vi "OP_Print_TPS20161121_cluster.vi"() -> ()   [LabVIEW 2013]
uses:
  <userlib>/caLab/Private/Get_PV-1D.vi
  <userlib>/caLab/Private/Get_PV.vi
panel:
  out "x = y?":bool
  out "NOW time":string
  out "NOW date":string
  out "loop2":i32=243
  in  "Save Button":bool
  out "error out 3":errorcluster
  in  "stop":bool
  out "time kickeron":string="kickers"
  out "date kickeron":string="wait to fire"
  out "Cluster":T1={"SR Fill Pattern"=array[864 elements], "Beam Current(mA"=301.91562200000004, "Beam Lifetime(min)"=669.1065769463743, "Beamsize X(um)"=55.54579477590784, "Beamsize Y(um)"=33.648665625479325, "Tune X(from BPM)"=0.1399, "Tune Y(from BPM)"=0.14, "Mode"="Top-Up", "NuX(from BBF) "=0.16718639681347974, "NuY(from BBF)"=0.25219386232318686, "IU22-23gap(R)"=11.0, "IU22-05gap(R)"=7.558, "IU22-05M"=TRUE, "IU22A-09gap(R)"=8.075, "IU22A-09M"=TRUE, "IU22B-09gap(R)"=40.001, "IU22B-09M"=FALSE, "IUT22-21gap(R)"=7.0, "IUT22-21M"=TRUE, "IU22-23M"=TRUE, "IU22A-25gap(R)"=8.18, "IU22A-25M"=TRUE, "IU22B-25gap(R)"=40.0, "IU22B-25M"=FALSE, "EPU48A-41gap(R)"=64.99985000000001, "EPU48A-41gM"=TRUE, "EPU48B-41gap(R)"=65.00399999999999, "EPU48B-41gM"=FALSE, "EPU46-45gap(R)"=45.00005, "EPU46-45gM"=TRUE, "EPU48A-41phase(R)"=0.0001, "EPU48B-41phase(R)"=0.00055, "EPU46-45phase(R)"=0.0, "Grid volt.(V)(S)"=33.0, "Gun mode"="MBM", "Mod.3 HV(kV)(S)"=35.800000000000026, "SR"="SR_DMB_2016_1102_1124LOCO.data", "BR"="Booster_JT_2016_1005_1200.data", "Linac"="Linac2016_1005_0935.data", "LTB"="LTB_JT_2016_1005_1200.data", "BTS"="BTS_2016_1116_1020.data", "RF2 remote"=TRUE, "RF2 OP mode"=TRUE, "RF2 phase.(S)"=-56.70000000000001, "RF Freq.(s)"=499654660.62238467, "RF2 gap volt.(S)"=1400.0, "RF3 remote"=TRUE, "RF3 OP mode"=TRUE, "RF3 phase.(S)"=160.0, "RF3 gap volt.(S)"=1400.0, "BBF V"=TRUE, "BBF H"=TRUE, "BR ext. kicker1(kV)"=18.266, "BR ext. kicker2(kV)"=18.26600000000001, "BR ext. sep.1(V)"=318.8444, "BR ext. sep.2(V)"=444.5, "BR inj. sep.(V)"=105.2, "BR inj. kicker(kV)"=16.40000000000001, "SR kicker4(kV)"=8.27, "SR kicker3(kV)"=8.315, "SR kicker2(kV)"=8.325, "SR kicker1(kV)"=8.4, "SR inj. sep.2(V)"=417.0, "SR inj. sep.1(V)"=419.3416, "Bucket Start"=100.0, "Bucket Last"=630.0, "Bucket Step"=10.0, "Orbit ILK(P)"=TRUE, "IU22-05 Hutch Enable"=TRUE, "IU22A-09M Hutch Enable"=TRUE, "IUT22-21M Hutch Enable"=TRUE, "IU22-23M Hutch Enable"=FALSE, "IU22A-25M Hutch Enable"=TRUE, "EPU48A-41M Hutch Enable"=FALSE, "EPU46-45M Hutch Enable"=TRUE, "EPU46-45 FE Enable"=TRUE, "EPU48A-41 FE Enable"=FALSE, "IU22A-25 FE Enable"=TRUE, "IU22-23 FE Enable"=FALSE, "IUT22-21 FE Enable"=TRUE, "IU22A-09 FE Enable"=TRUE, "IU22-05 FE Enable"=TRUE, "EPU48A-41pM"=TRUE, "EPU48B-41pM"=FALSE, "EPU46-45pM"=FALSE, "Gun volt.(V)(S)"=23.5, "Width count"=30.0, "2ns step"=0.0, "10ps delay"=100.0, "phase shifter"=130.00060000000002, "Taper"=-1.0899999999999999, "05XBPMX 1"=115.877, "09XBPMX 1"=471.421, "21XBPMX 1"=612.331, "23XBPMX 1"=-46.736000000000004, "25XBPMX 1"=462.29900000000004, "41XBPMX 1"=364.139, "45XBPMX 1"=-164.196, "05XBPMY 1"=-62.875, "09XBPMY 1"=-23.034, "21XBPMY 1"=-27.449, "23XBPMY 1"=-89.72200000000001, "25XBPMY 1"=459.291, "41XBPMY 1"=-111.624, "45XBPMY 1"=-57.689, "FOFB H"="On", "FOFB V"="On", "time string"="21:36:25", "date"="2016/11/21", "date (last kicker ON)"="wait to fire", "time string (last kicker ON)"="", "BPMX Graph"={[1, 2, 3, 4, 5, 6, 7, 8, 9, 10, 11, 12, 13, 14, 15, 16, 17, 18, 19, 20, 21, 22, 23, 24, 25, 26, 27, 28, 29, 30, 31, 32, 33, 34, 35, 36, 37, 38, 39, 40, 41, 42, 43, 44, 45, 46, 47, 48, 49, 50, 51, 52, 53, 54, 55, 56, 57, 58, 59, 60, 61, 62, 63, 64, 65, 66, 67, 68, 69, 70, 71, 72, 73, 74, 75, 76, 77, 78, 79, 80, 81, 82, 83, 84, 85, 86, 87, 88, 89, 90, 91, 92, 93, 94, 95, 96, 97, 98, 99, 100, 101, 102, 103, 104, 105, 106, 107, 108, 109, 110, 111, 112, 113, 114, 115, 116, 117, 118, 119, 120, 121, 122, 123, 124, 125, 126, 127, 128, 129, 130, 131, 132, 133, 134, 135, 136, 137, 138, 139, 140, 141, 142, 143, 144, 145, 146, 147, 148, 149, 150, 151, 152, 153, 154, 155, 156, 157, 158, 159, 160, 161, 162, 163, 164, 165, 166, 167, 168, 169, 170, 171, 172, 173, 174], "1rst Value (number)"=[-31.198, -3.303, -73.172, -2.032, 86.386, -75.851, 71.519, -46.03, 6.824, -37.804, 68.275, -4.672, -223.404, -16.867, -6.964, -259.448, -62.697, 1.8880000000000001, 75.267, -92.668, 86.714, -30.843, 12.767, -107.398, -44.436, 161.126, 208.922, 211.488, -27.247, 79.489, 826.962, 470.705, -115.522, -41.497, 159.486, -54.261, -0.64, 42.641, -2.466, -143.394, -24.785, 138.912, -65.805, 42.325, 32.891, -7.298, -96.724, -31.725, 98.531, -80.64, 64.163, 94.83, -44.03, -163.192, 50.589, 46.669000000000004, -87.508, 78.479, 31.618000000000002, -17.077, -125.32600000000001, -3.845, 98.34100000000001, -39.679, 50.247, -58.208, 40.297000000000004, -69.857, 42.548, -19.403, -211.0, -9.082, -322.597, -233.847, -140.75, 97.087, -15.869, -29.053, 59.46, -115.316, 70.896, -60.685, 33.715, 12.09, -520.422, -138.423, -302.753, 79.862, 120.014, 122.671, -55.812, 27.084, 39.115, -138.936, 156.631, 53.777, -72.647, -52.588, 16.002, 45.197, -117.489, 121.709, 27.952, -31.609, -113.58500000000001, 45.019, 55.136, -130.553, 138.93200000000002, 35.998, -30.631, -96.529, -7.589, 100.395, -93.919, 40.569, 79.538, -68.044, -134.578, 2.52, 84.539, -59.166000000000004, 42.576, 34.657000000000004, -15.805, -52.158, 18.484, 4.346, -157.404, 182.672, 202.518, -164.868, -53.871, 8.066, -9.738, -55.594, 92.623, -13.785, 11.587, -60.627, -47.704, 65.516, 57.924, 148.347, -201.348, -302.753, 189.117, 72.681, -134.928, 39.791000000000004, 45.938, -49.072, 54.473, 28.991, -20.657, -80.283, -20.264, 106.907, -121.271, 150.281, -2.243, -11.844, -122.82300000000001, 0.973, 114.186, -107.94, 95.485, 40.314, -36.956, -134.537, 16.196, 91.88, -35.505, -0.018000000000000002]}, "BPMY Graph"={[1, 2, 3, 4, 5, 6, 7, 8, 9, 10, 11, 12, 13, 14, 15, 16, 17, 18, 19, 20, 21, 22, 23, 24, 25, 26, 27, 28, 29, 30, 31, 32, 33, 34, 35, 36, 37, 38, 39, 40, 41, 42, 43, 44, 45, 46, 47, 48, 49, 50, 51, 52, 53, 54, 55, 56, 57, 58, 59, 60, 61, 62, 63, 64, 65, 66, 67, 68, 69, 70, 71, 72, 73, 74, 75, 76, 77, 78, 79, 80, 81, 82, 83, 84, 85, 86, 87, 88, 89, 90, 91, 92, 93, 94, 95, 96, 97, 98, 99, 100, 101, 102, 103, 104, 105, 106, 107, 108, 109, 110, 111, 112, 113, 114, 115, 116, 117, 118, 119, 120, 121, 122, 123, 124, 125, 126, 127, 128, 129, 130, 131, 132, 133, 134, 135, 136, 137, 138, 139, 140, 141, 142, 143, 144, 145, 146, 147, 148, 149, 150, 151, 152, 153, 154, 155, 156, 157, 158, 159, 160, 161, 162, 163, 164, 165, 166, 167, 168, 169, 170, 171, 172, 173, 174], "1rst Value (number)"=[-99.743, 2.851, -30.024, 83.777, -46.733000000000004, -39.889, 2.349, -4.944, 17.022000000000002, 9.824, 11.632, 41.188, -13.992, 13.911, -6.211, 53.857, -48.993, -32.789, -6.3740000000000006, -62.867000000000004, -8.332, 72.09400000000001, -75.398, 53.283, 63.008, -2.23, 43.024, 32.073, -246.641, -93.162, 456.41700000000003, 88.299, 58.803000000000004, 1.7590000000000001, 35.664, 6.575, 18.59, -30.439, 11.254, -28.256, -62.707, -4.503, 1.31, -21.571, 34.77, -8.876, 31.237000000000002, 25.402, 2.726, 20.655, -7.845, -1.443, -31.935000000000002, -16.981, 13.022, 17.515, -82.867, 61.285000000000004, -57.573, 110.363, -27.753, 28.322, -9.241, 53.929, -25.816, 24.231, -57.876, -11.578, 32.087, -70.84, 64.43, 9.409, -157.639, -57.0, 39.267, 30.23, 18.993000000000002, -33.97, 26.195, -10.585, -17.617, -18.667, 31.615000000000002, -25.437, 29.564, 13.537, 6.728, 163.38400000000001, 106.51, -70.056, 12.874, -4.125, -10.855, -21.856, 1.947, 8.096, 11.402000000000001, 5.761, 41.929, -8.752, 18.634, 7.553, -40.034, 39.183, -25.067, -32.557, 5.393, -17.564, -1.614, 20.498, -14.818, 10.313, 35.254, -35.886, 58.359, -36.56, -20.354, 7.593, -21.256, -8.001, -16.79, 10.18, -16.327, 20.416, -10.539, 19.944, -6.801, 13.068, -13.644, 3.468, -0.983, -17.6, 6.785, -26.101, -11.52, 61.191, -32.777, 13.536, 4.026, -14.682, 52.057, -53.883, 27.118000000000002, 31.672, 79.62, 17.715, 15.693, 113.157, -57.095, 14.214, -4.787, -11.148, -3.157, -6.251, -0.764, 3.563, 7.3500000000000005, 10.779, 21.129, 11.36, 7.771, -14.787, -13.278, 0.279, -13.516, -62.422000000000004, -13.389000000000001, 80.56400000000001, -108.465, 69.885, 30.116, 21.421, 32.779, -10.527000000000001]}, "Radio Buttons 2"=enum."absolute"} {"45XBPMY 1" format="%#.2f"; "41XBPMY 1" format="%#.2f"; "25XBPMY 1" format="%#.2f"; "23XBPMY 1" format="%#.2f"; "21XBPMY 1" format="%#.2f"; "09XBPMY 1" format="%#.2f"; "05XBPMY 1" format="%#.2f"; "45XBPMX 1" format="%#.2f"; "41XBPMX 1" format="%#.2f"; "25XBPMX 1" format="%#.2f"; "23XBPMX 1" format="%#.2f"; "21XBPMX 1" format="%#.2f"; "09XBPMX 1" format="%#.2f"; "05XBPMX 1" format="%#.2f"; "Taper" format="%#.4f"; "phase shifter" format="%#.3f"; "10ps delay" format="%#.1f"; "2ns step" format="%#.1f"; "Width count" format="%#.1f"; "Gun volt.(V)(S)" format="%#.1f"; "Bucket Step" format="%#.2f"; "Bucket Last" format="%#.2f"; "Bucket Start" format="%#.2f"; "BR ext. kicker1(kV)" format="%#.2f"; "BR ext. kicker2(kV)" format="%#.2f"; "BR ext. sep.1(V)" format="%#.2f"; "BR ext. sep.2(V)" format="%#.2f"; "BR inj. sep.(V)" format="%#.3f"; "BR inj. kicker(kV)" format="%#.3f"; "SR kicker4(kV)" format="%#.2f"; "SR kicker3(kV)" format="%#.2f"; "SR kicker2(kV)" format="%#.2f"; "SR kicker1(kV)" format="%#.2f"; "SR inj. sep.2(V)" format="%#.2f"; "SR inj. sep.1(V)" format="%#.2f"; "RF3 gap volt.(S)" format="%#.0f"; "RF3 phase.(S)" format="%#.1f"; "RF2 gap volt.(S)" format="%#.0f"; "RF Freq.(s)" format="%#.1f"; "RF2 phase.(S)" format="%#.1f"; "Mod.3 HV(kV)(S)" format="%#.3f"; "Grid volt.(V)(S)" format="%#.1f"; "EPU46-45phase(R)" format="%#.4f"; "EPU48B-41phase(R)" format="%#.4f"; "EPU48A-41phase(R)" format="%#.4f"; "EPU46-45gap(R)" format="%#.4f"; "EPU48B-41gap(R)" format="%#.4f"; "EPU48A-41gap(R)" format="%#.4f"; "IU22B-25gap(R)" format="%#.4f"; "IU22A-25gap(R)" format="%#.4f"; "IUT22-21gap(R)" format="%#.4f"; "IU22B-09gap(R)" format="%#.4f"; "IU22A-09gap(R)" format="%#.4f"; "IU22-05gap(R)" format="%#.4f"; "IU22-23gap(R)" format="%#.4f"; "NuY(from BBF)" format="%#.4f"; "NuX(from BBF)" format="%#.4f"; "Tune Y(from BPM)" format="%#.4f"; "Tune X(from BPM)" format="%#.4f"; "Beamsize Y(um)" format="%#.2f"; "Beamsize X(um)" format="%#.2f"; "Beam Lifetime(min)" format="%#.3f"; "Beam Current(mA" format="%#.3f"}
  out "date (last Gun ON)":string="2016/08/29"
  out "time string (last Gun ON)":string="23:28:50"
  out "Value Array (number) 7":dbl[](array[numeric])=[115.877, -62.875, 471.421, -23.034, 612.331, -27.449, -46.736000000000004, -89.72200000000001, 462.29900000000004, 459.291, 364.139, -111.624, -164.196, -57.689]
  out "Value Array (number) 6":dbl[](array[numeric])=[7.558, 8.075, 40.001, 7.0, 11.0, 8.18, 40.0, 64.99985000000001, 0.0001, 65.00399999999999, 0.00055, 45.00005, 0.0, -1.0899999999999999, 130.00060000000002]
  out "1rst Value (string) 2":string[](array[string])=["MBM", "33", "23.5", "350", "35.8", "22485", "22485", "62", "30", "0", "0", "160", "100"]
  out "Value Array (number) 5":dbl[](array[numeric])=[499654641.19275105, 1.0, 0.0, 1335.005102558433, 1400.0, -56.1, 1.0, 0.0, 1362.1066276040413, 1400.0, 160.0]
  out "1rst Value (string)":string[](array[string])=["Linac2016_1005_0935.data", "LTB_JT_2016_1005_1200.data", "Booster_JT_2016_1005_1200.data", "BTS_2016_1116_1020.data", "SR_DMB_2016_1102_1124LOCO.data"]
  out "Value Array (number) 4":dbl[](array[numeric])=[499654660.62238467, 1.0, 0.0, 1334.266859115235, 1400.0, -56.70000000000001, 1.0, 0.0, 1364.570619451613, 1400.0, 160.0]
  out "Value Array (number) 3":dbl[](array[numeric])=[0.0, 33.0, 23.5, 350.0, 35.800000000000026, 22485.0, 22485.0, 62.0, 30.0, 0.0, 0.0, 160.0, 100.0]
  out "Value Array (number) 2":dbl[](array[numeric])=[105.2, 16.40000000000001, 18.266, 18.26600000000001, 318.8444, 444.5, 419.3416, 417.0, 8.4, 8.325, 8.315, 8.27]
  out "Value Array (number)":dbl[](array[numeric])=[1.0, 301.91562200000004, 669.1065769463743, 46.211143740355936, 27.993898190914578, 0.11937377690802348, 0.2162426614481409, 96.68439483642578, 145.84446716308594, 100.0, 630.0, 10.0]
  out "Orbit ILK(A)":bool
  out "Orbit INT. Ang Active":bool
  out "Orbit INT.Ang. On":bool
  out "Orbit INT. Pos Active":bool
  out "Orbit INT.Pos. On":bool
  out "SBM volt.(S)":dbl=350.0 format="%#.1f"
  out "MBM volt.(S)":dbl=23.5 format="%#.1f"
  in  "Copy Button":bool
  in  "Print Button":bool
  in  "Help Button":bool
  in  "Refresh Button":bool
  in  "Open Button":bool
  out "Gun WCM":dbl[](graph)
  out "BR Fill Pattern":dbl[](graph)
  # "TPS OP Handover Information"
  # "Others"
  # "Time："
  # "Valve  Status"
  # "SM Status"
  # "歷史電流圖\ntrip次數?\n輻射劑量?\n平均氣壓\n目前最高累計劑量\n最近一次觸發時BR電流及WCM數值"
  # "TPS Operational Handover Information v1.0"
  # "SR Status"
  # "Feedback"
  # "Pulse Mag"
  # "LINAC"
  # "x8(ns)"
  # "x2(ns)"
  # "x0.01(ns)"
  # "RF Status"
  # "Hz"
  # "(kV)"
  # "(kV)"
  # "Changeliang@LOP.NSRRC"
  # "SR Fill Pattern"
  # "Lattice Files in using"
  # "ID &Beamline (R)"
  # "Gap\nmm"
  # "Motor"
  # "Phase"
  # "FE/Hutch"
  # "phase\nshifter"
  # "Taper\n(enc)"
  # "XBPM1X\num"
  # "XBPM1Y\num"
  # "05"
  # "09"
  # "21"
  # "23"
  # "25"
  # "41"
  # "45"
  # "SR Orbit"
  # "BPMX"
  # "BPMY"
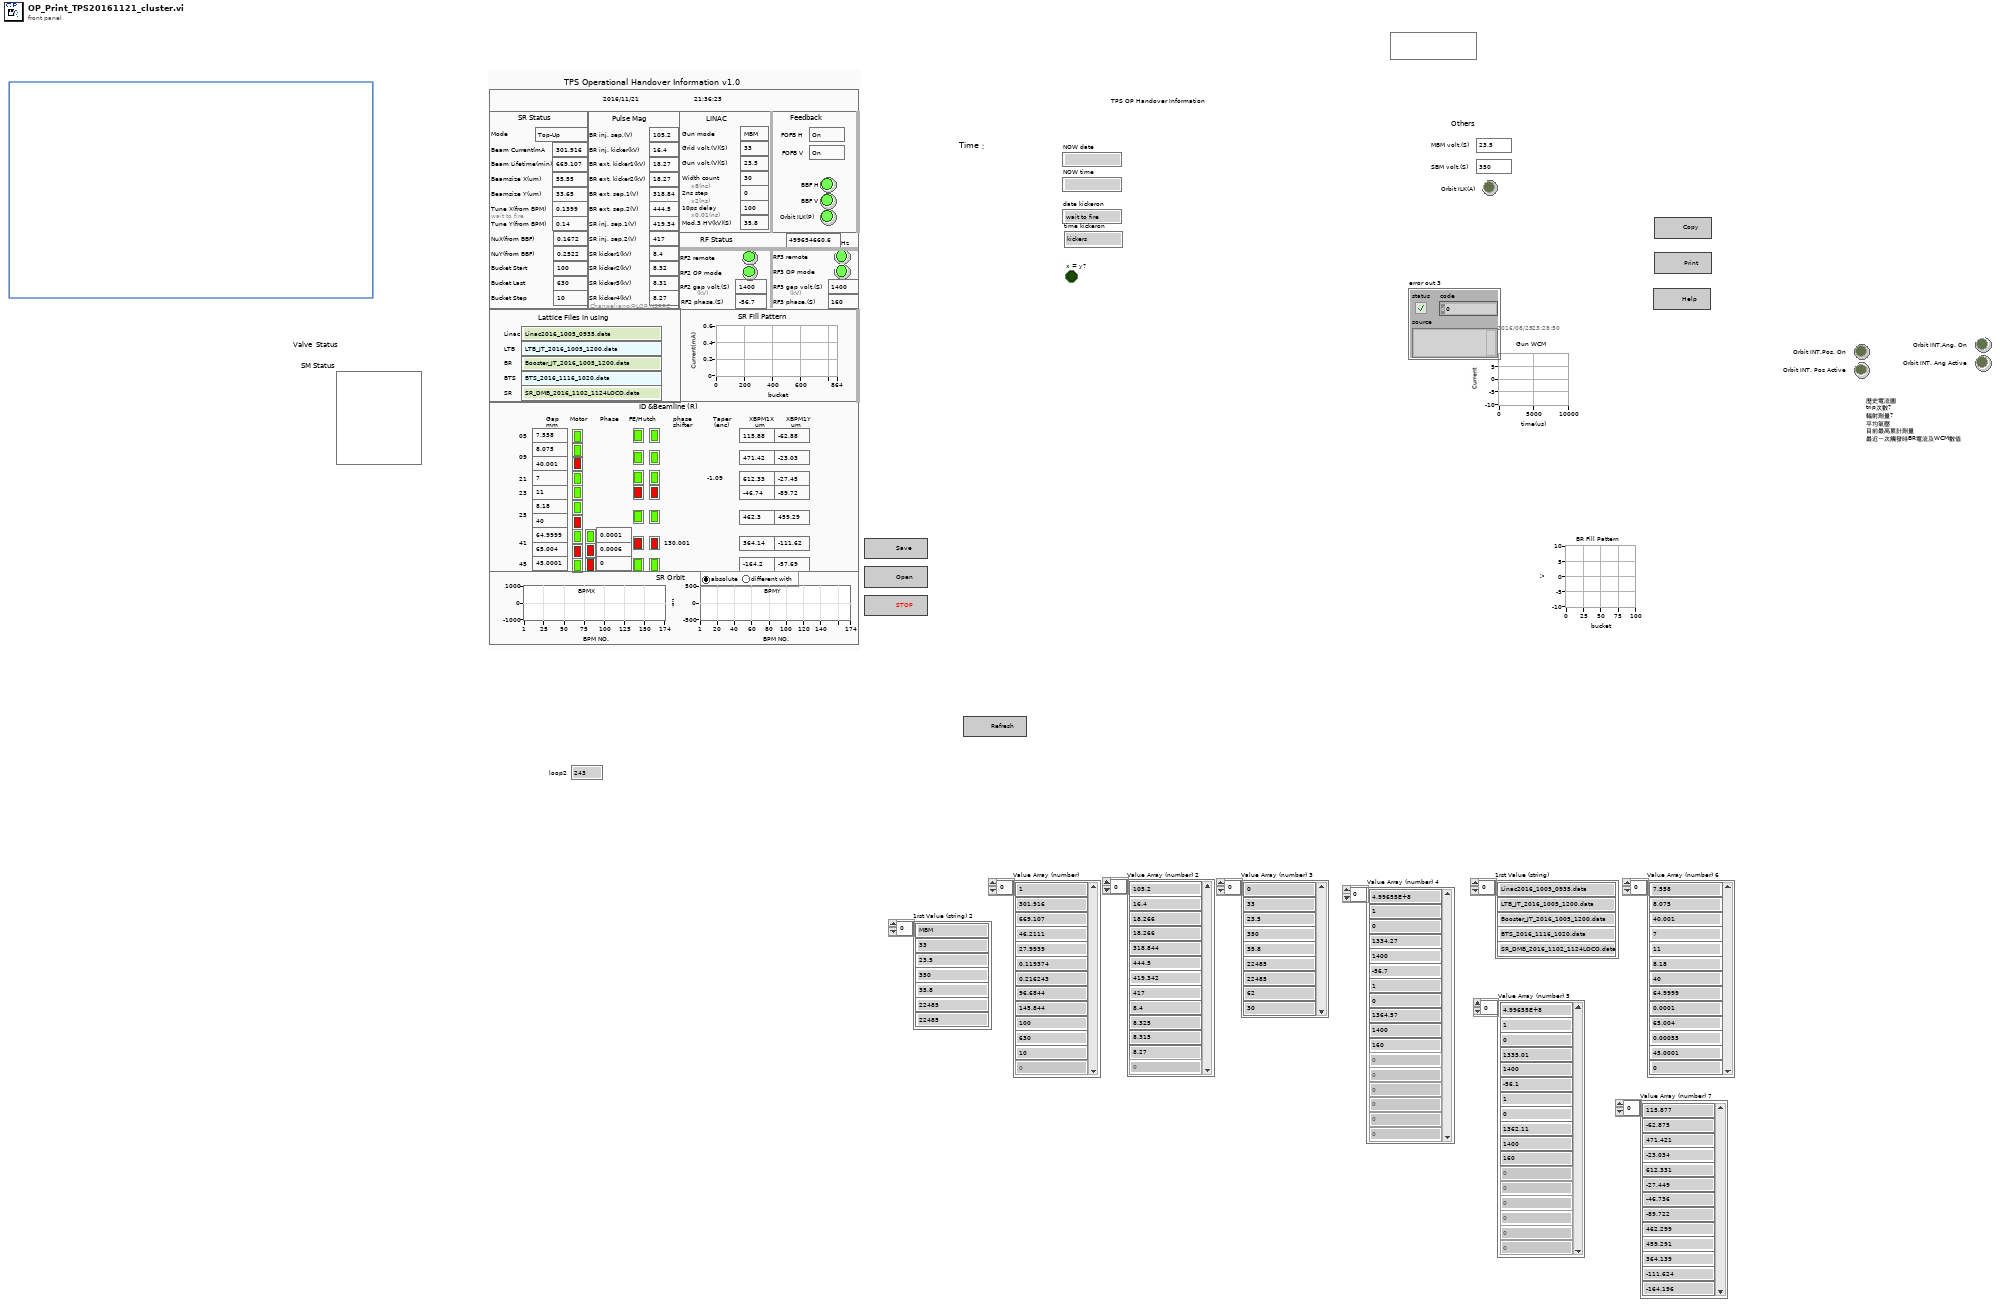
[diagram p1: front panel]
types:
  T1 = cluster{"SR Fill Pattern":dbl[], "Beam Current(mA":dbl, "Beam Lifetime(min)":dbl, "Beamsize X(um)":dbl, "Beamsize Y(um)":dbl, "Tune X(from BPM)":dbl, "Tune Y(from BPM)":dbl, "Mode":string, "NuX(from BBF) ":dbl, "NuY(from BBF)":dbl, "IU22-23gap(R)":dbl, "IU22-05gap(R)":dbl, "IU22-05M":bool, "IU22A-09gap(R)":dbl, "IU22A-09M":bool, "IU22B-09gap(R)":dbl, "IU22B-09M":bool, "IUT22-21gap(R)":dbl, "IUT22-21M":bool, "IU22-23M":bool, "IU22A-25gap(R)":dbl, "IU22A-25M":bool, "IU22B-25gap(R)":dbl, "IU22B-25M":bool, "EPU48A-41gap(R)":dbl, "EPU48A-41gM":bool, "EPU48B-41gap(R)":dbl, "EPU48B-41gM":bool, "EPU46-45gap(R)":dbl, "EPU46-45gM":bool, "EPU48A-41phase(R)":dbl, "EPU48B-41phase(R)":dbl, "EPU46-45phase(R)":dbl, "Grid volt.(V)(S)":dbl, "Gun mode":string, "Mod.3 HV(kV)(S)":dbl, "SR":string, "BR":string, "Linac":string, "LTB":string, "BTS":string, "RF2 remote":bool, "RF2 OP mode":bool, "RF2 phase.(S)":dbl, "RF Freq.(s)":dbl, "RF2 gap volt.(S)":dbl, "RF3 remote":bool, "RF3 OP mode":bool, "RF3 phase.(S)":dbl, "RF3 gap volt.(S)":dbl, "BBF V":bool, "BBF H":bool, "BR ext. kicker1(kV)":dbl, "BR ext. kicker2(kV)":dbl, "BR ext. sep.1(V)":dbl, "BR ext. sep.2(V)":dbl, "BR inj. sep.(V)":dbl, "BR inj. kicker(kV)":dbl, "SR kicker4(kV)":dbl, "SR kicker3(kV)":dbl, "SR kicker2(kV)":dbl, "SR kicker1(kV)":dbl, "SR inj. sep.2(V)":dbl, "SR inj. sep.1(V)":dbl, "Bucket Start":dbl, "Bucket Last":dbl, "Bucket Step":dbl, "Orbit ILK(P)":bool, "IU22-05 Hutch Enable":bool, "IU22A-09M Hutch Enable":bool, "IUT22-21M Hutch Enable":bool, "IU22-23M Hutch Enable":bool, "IU22A-25M Hutch Enable":bool, "EPU48A-41M Hutch Enable":bool, "EPU46-45M Hutch Enable":bool, "EPU46-45 FE Enable":bool, "EPU48A-41 FE Enable":bool, "IU22A-25 FE Enable":bool, "IU22-23 FE Enable":bool, "IUT22-21 FE Enable":bool, "IU22A-09 FE Enable":bool, "IU22-05 FE Enable":bool, "EPU48A-41pM":bool, "EPU48B-41pM":bool, "EPU46-45pM":bool, "Gun volt.(V)(S)":dbl, "Width count":dbl, "2ns step":dbl, "10ps delay":dbl, "phase shifter":dbl, "Taper":dbl, "05XBPMX 1":dbl, "09XBPMX 1":dbl, "21XBPMX 1":dbl, "23XBPMX 1":dbl, "25XBPMX 1":dbl, "41XBPMX 1":dbl, "45XBPMX 1":dbl, "05XBPMY 1":dbl, "09XBPMY 1":dbl, "21XBPMY 1":dbl, "23XBPMY 1":dbl, "25XBPMY 1":dbl, "41XBPMY 1":dbl, "45XBPMY 1":dbl, "FOFB H":string, "FOFB V":string, "time string":string, "date":string, "date (last kicker ON)":string, "time string (last kicker ON)":string, "BPMX Graph":cluster{i32[], "1rst Value (number)":dbl[]}, "BPMY Graph":cluster{i32[], "1rst Value (number)":dbl[]}, "Radio Buttons 2":enum32{"absolute", "different with"}}
  T2 = cluster{"SR Fill Pattern":dbl[], "Beam Current(mA":dbl, "Beam Lifetime(min)":dbl, "Beamsize X(um)":dbl, "Beamsize Y(um)":dbl, "Tune X(form BPM)":dbl, "Tune Y(form BPM)":dbl, "Mode":string, "NuX(form BBF) ":dbl, "NuY(form BBF)":dbl, "IU22-23gap(R)":dbl, "IU22-05gap(R)":dbl, "IU22-05M":bool, "IU22A-09gap(R)":dbl, "IU22A-09M":bool, "IU22B-09gap(R)":dbl, "IU22B-09M":bool, "IUT22-21gap(R)":dbl, "IUT22-21M":bool, "IU22-23M":bool, "IU22A-25gap(R)":dbl, "IU22A-25M":bool, "IU22B-25gap(R)":dbl, "IU22B-25M":bool, "EPU48A-41gap(R)":dbl, "EPU48A-41gM":bool, "EPU48B-41gap(R)":dbl, "EPU48B-41gM":bool, "EPU46-45gap(R)":dbl, "EPU46-45gM":bool, "EPU48A-41phase(R)":dbl, "EPU48B-41phase(R)":dbl, "EPU46-45phase(R)":dbl, "Grid volt.(S)":dbl, "Gun mode":string, "Mod.3 HV(S)":dbl, "SR":string, "BR":string, "Linac":string, "LTB":string, "BTS":string, "RF2 remote":bool, "RF2 OP mode":bool, "RF2 phase.(S)":dbl, "RF Freq.(s)":dbl, "RF2 gap volt.(S)":dbl, "RF3 remote":bool, "RF3 OP mode":bool, "RF3 phase.(S)":dbl, "RF3 gap volt.(S)":dbl, "BBF V":bool, "BBF H":bool, "BR ext. kicker1":dbl, "BR ext. kicker2":dbl, "BR ext. sep.1":dbl, "BR ext. sep.2":dbl, "BR inj. sep.":dbl, "BR inj. kicker":dbl, "SR kicker4":dbl, "SR kicker3":dbl, "SR kicker2":dbl, "SR kicker1":dbl, "SR inj. sep.2":dbl, "SR inj. sep.1":dbl, "Bucket Start":dbl, "Bucket Last":dbl, "Bucket Step":dbl, "Orbit ILK(P)":bool, "IU22-05 Hutch Enable":bool, "IU22A-09M Hutch Enable":bool, "IUT22-21M Hutch Enable":bool, "IU22-23M Hutch Enable":bool, "IU22A-25M Hutch Enable":bool, "EPU48A-41M Hutch Enable":bool, "EPU46-45M Hutch Enable":bool, "EPU46-45 FE Enable":bool, "EPU48A-41 FE Enable":bool, "IU22A-25 FE Enable":bool, "IU22-23 FE Enable":bool, "IUT22-21 FE Enable":bool, "IU22A-09 FE Enable":bool, "IU22-05 FE Enable":bool, "EPU48A-41pM":bool, "EPU48B-41pM":bool, "EPU46-45pM":bool, "Gun volt.(S)":dbl, "Width count":dbl, "2ns step":dbl, "10ps delay":dbl, "phase shifter":dbl, "Taper":dbl, "05XBPMX 1":dbl, "09XBPMX 1":dbl, "21XBPMX 1":dbl, "23XBPMX 1":dbl, "25XBPMX 1":dbl, "41XBPMX 1":dbl, "45XBPMX 1":dbl, "05XBPMY 1":dbl, "09XBPMY 1":dbl, "21XBPMY 1":dbl, "23XBPMY 1":dbl, "25XBPMY 1":dbl, "41XBPMY 1":dbl, "45XBPMY 1":dbl, "FOFB H":string, "FOFB V":string, "time string":string, "date":string, "date (last kicker ON)":string, "time string (last kicker ON)":string, "BPMX Graph":cluster{i32[], "1rst Value (number)":dbl[]}, "BPMY Graph":cluster{i32[], "1rst Value (number)":dbl[]}, "Radio Buttons 2":enum32{"absolute", "different with"}}
  T3 = typedef "imagedata.ctl" = cluster{"image type":i32, "image depth":i32, "image":u8[], "mask":u8[], "colors":u32[], "Rectangle":cluster{"left":i16, "top":i16, "right":i16, "bottom":i16}}
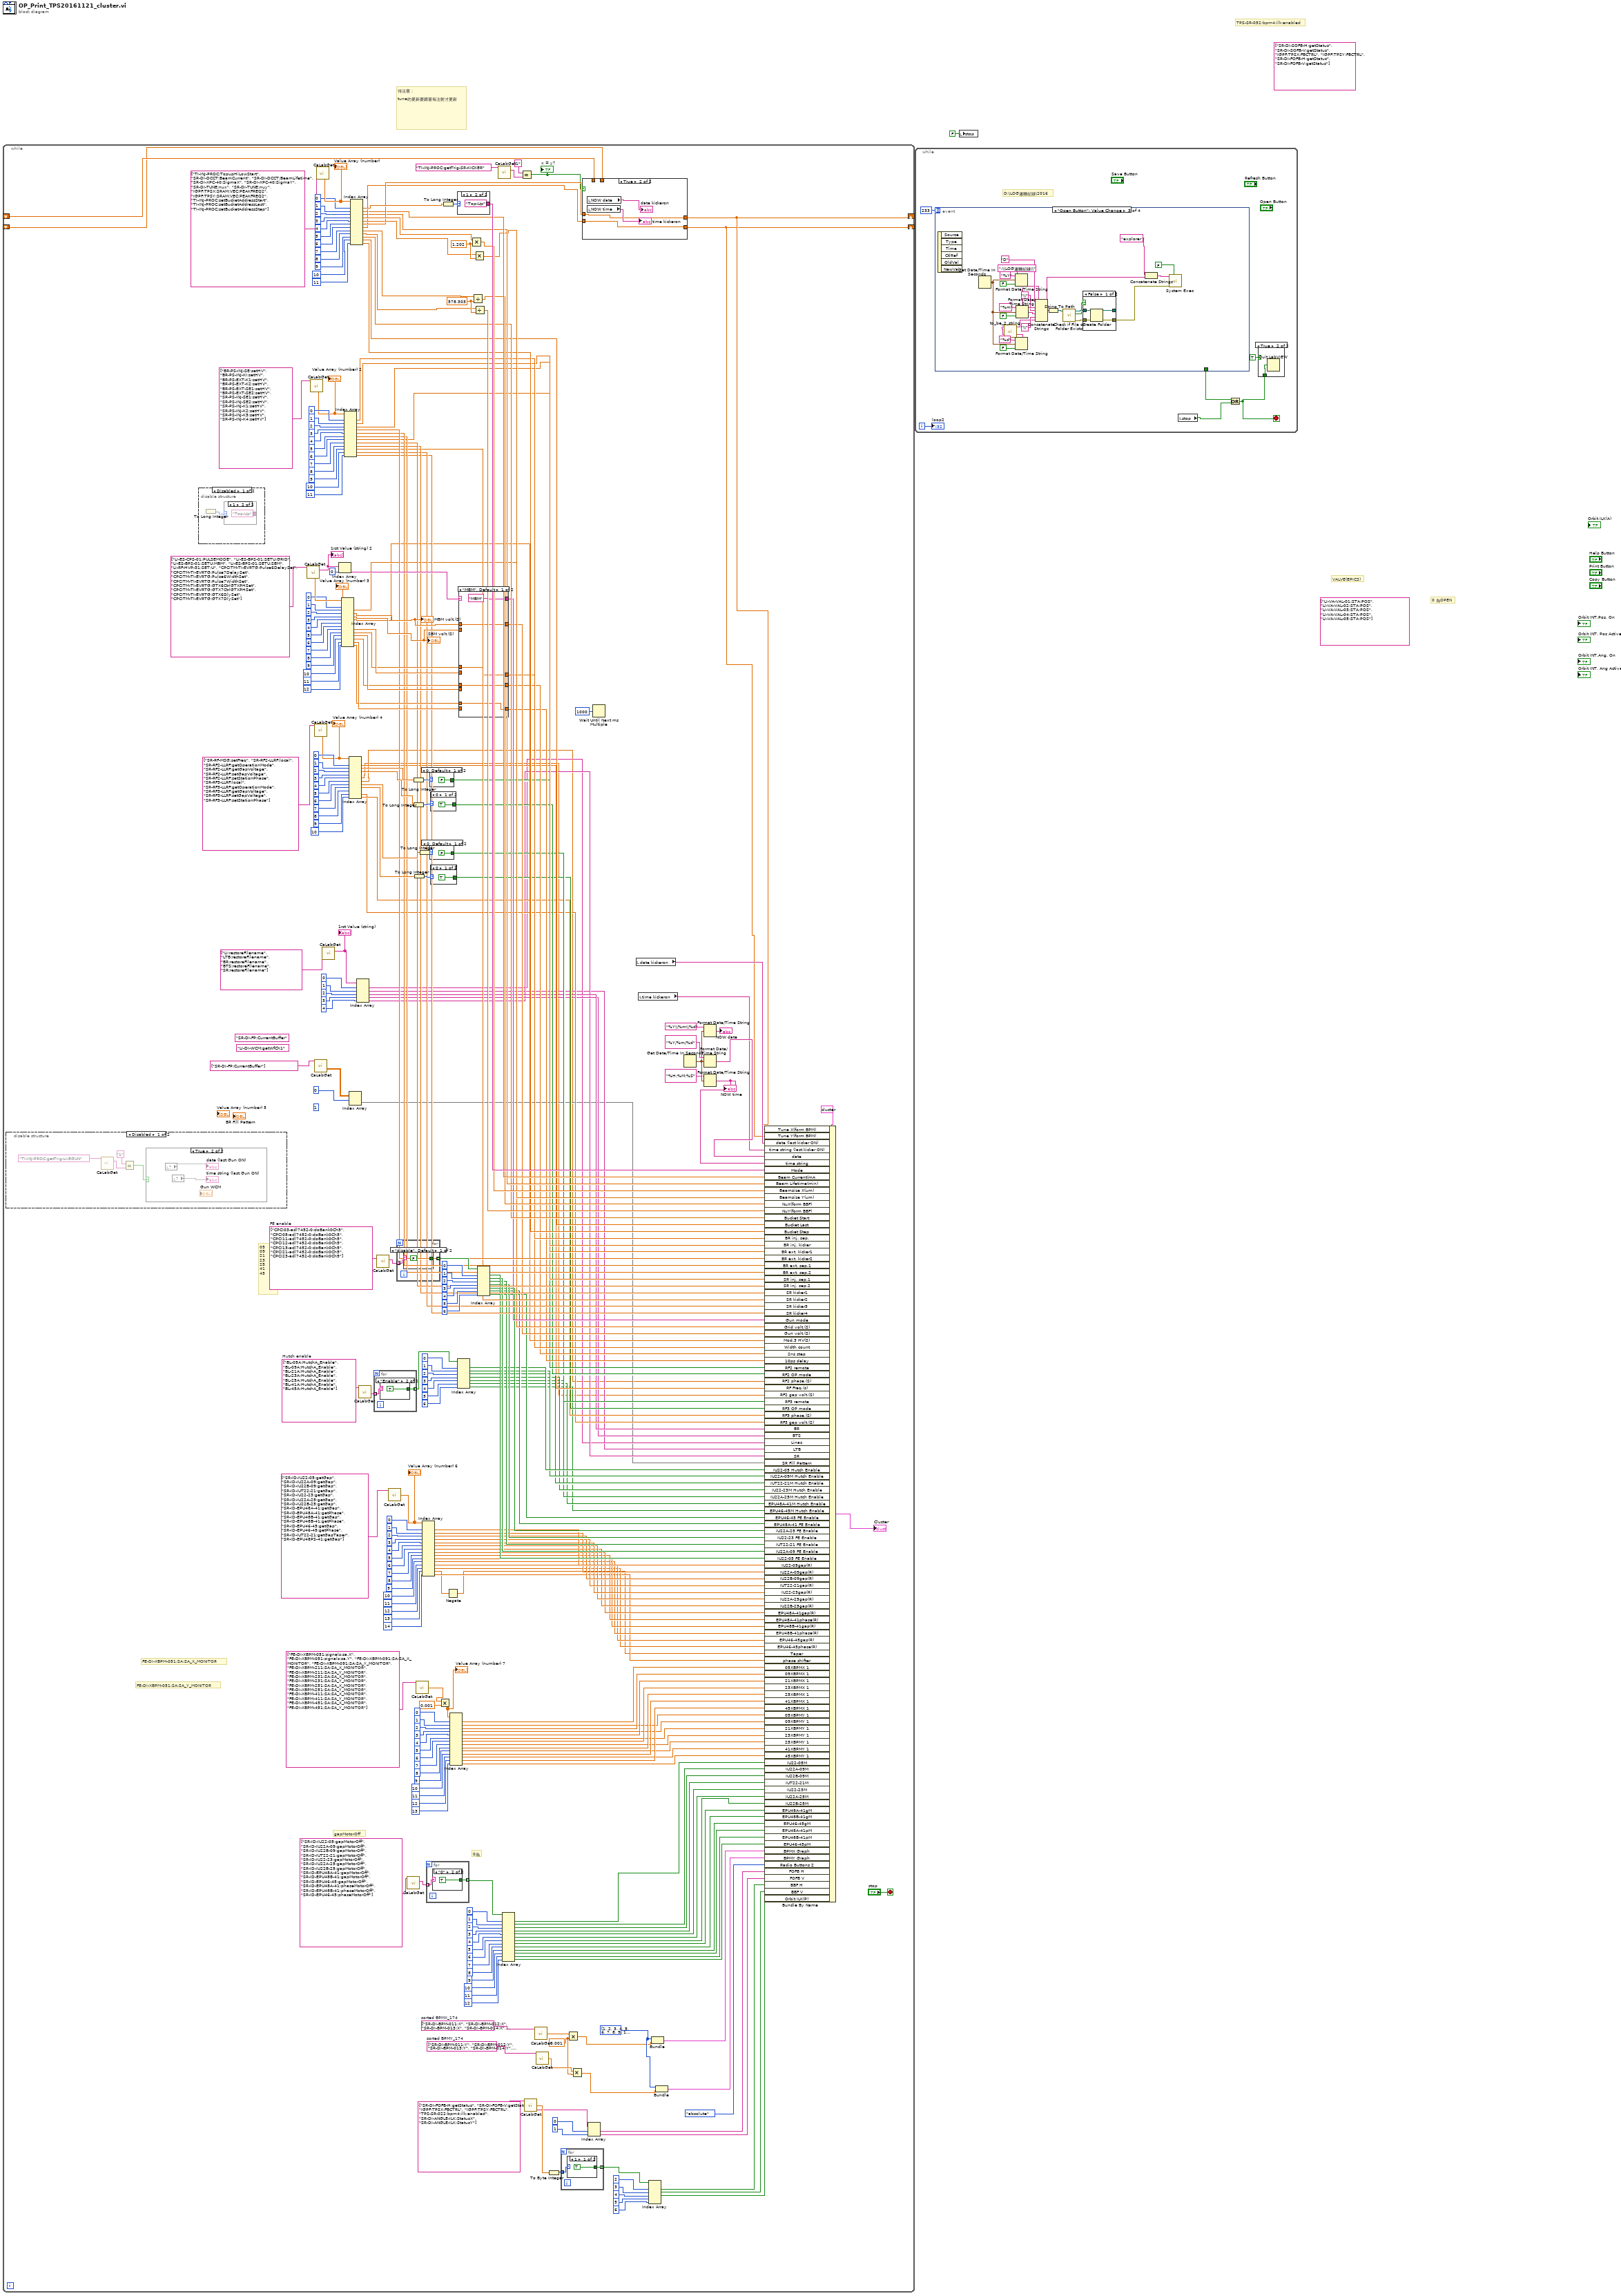
[diagram p0: block diagram]
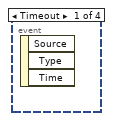
[diagram p3: hidden frame]
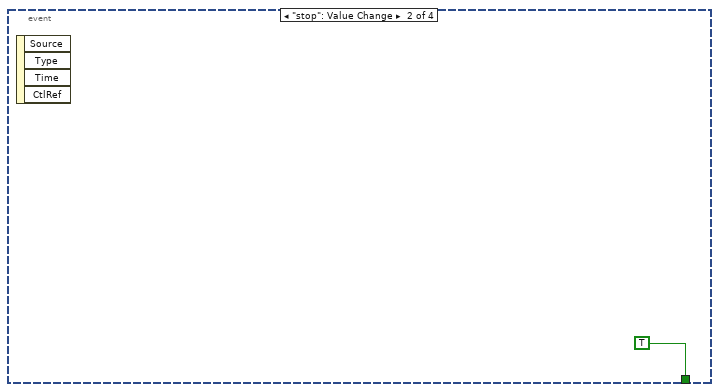
[diagram p4: hidden frame]
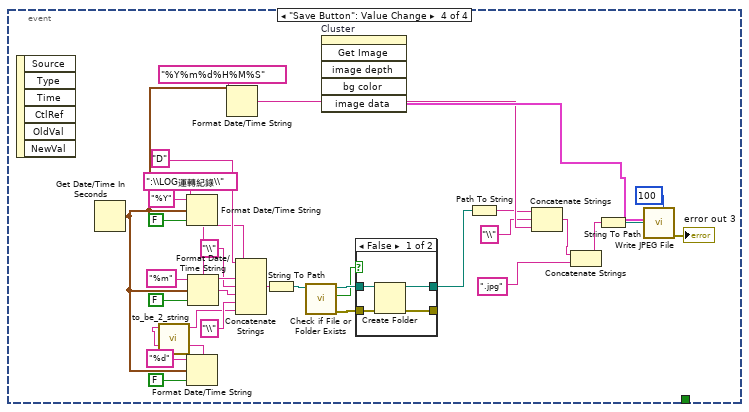
[diagram p6: hidden frame]
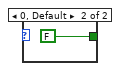
[diagram p8: hidden frame]
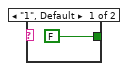
[diagram p11: hidden frame]
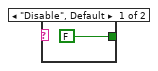
[diagram p12: hidden frame]
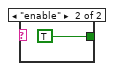
[diagram p13: hidden frame]
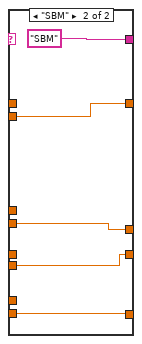
[diagram p14: hidden frame]
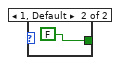
[diagram p16: hidden frame]
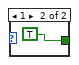
[diagram p17: hidden frame]
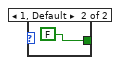
[diagram p18: hidden frame]
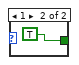
[diagram p19: hidden frame]
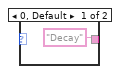
[diagram p20: hidden frame]
diagram:
  (unwired) string[] ["LI-VA-VAL-01:STA:POS", "LI-VA-VAL-02:STA:POS", "LI-VA-VAL-03:STA:POS", "LI-VA-VAL-04:STA:POS", "LI-VA-VAL-05:STA:POS"]
  (unwired) string[] ["SR-DI-SOFB-H:getStatus", "SR-DI-SOFB-V:getStatus", "IGPF:TPSX:FBCTRL", "IGPF:TPSY:FBCTRL", "SR-DI-FOFB-H:getStatus", "SR-DI-FOFB-V:getStatus"]
  # "TPS-SR-052:bpm4:ilk:enabled"
  # "待注意：\n\ntune的更新要跟著有注射才更新"
  # "0 為OPEN"
  # "VALVE(EPICS)"
  n1 = while {
    shift-right: [w5] -> _
    shift-left: _ -> [w3]
    shift-right: [w4] -> _
    shift-left: _ -> [w2]
    stop <- "stop" stop-if-true
    (unwired) "LI-DI-WCM:getWfCh1"
    (unwired) "SR-DI-FP:CurrentBuffer"
    w143 = i32[] [1, 2, 3, 4, 5, 6, 7, 8, 9, 10, 11, 12, 13, 14, 15, 16, 17, 18, 19, 20, 21, 22, 23, 24, 25, 26, 27, 28, 29, 30, 31, 32, 33, 34, 35, 36, 37, 38, 39, 40, 41, 42, 43, 44, 45, 46, 47, 48, 49, 50, 51, 52, 53, 54, 55, 56, 57, 58, 59, 60, 61, 62, 63, 64, 65, 66, 67, 68, 69, 70, 71, 72, 73, 74, 75, 76, 77, 78, 79, 80, 81, 82, 83, 84, 85, 86, 87, 88, 89, 90, 91, 92, 93, 94, 95, 96, 97, 98, 99, 100, 101, 102, 103, 104, 105, 106, 107, 108, 109, 110, 111, 112, 113, 114, 115, 116, 117, 118, 119, 120, 121, 122, 123, 124, 125, 126, 127, 128, 129, 130, 131, 132, 133, 134, 135, 136, 137, 138, 139, 140, 141, 142, 143, 144, 145, 146, 147, 148, 149, 150, 151, 152, 153, 154, 155, 156, 157, 158, 159, 160, 161, 162, 163, 164, 165, 166, 167, 168, 169, 170, 171, 172, 173, 174] ("Array 4")
    w140 = 0.001
    w137 = string[] ["SR-DI-BPM-011:Y", "SR-DI-BPM-012:Y", "SR-DI-BPM-013:Y", "SR-DI-BPM-014:Y", "SR-DI-BPM-015:Y", "SR-DI-BPM-016:Y", "SR-DI-BPM-017:Y", "SR-DI-BPM-021:Y", "SR-DI-BPM-022:Y", "SR-DI-BPM-023:Y", "SR-DI-BPM-024:Y", "SR-DI-BPM-025:Y", "SR-DI-BPM-026:Y", "SR-DI-BPM-027:Y", "SR-DI-BPM-031:Y", "SR-DI-BPM-032:Y", "SR-DI-BPM-033:Y", "SR-DI-BPM-034:Y", "SR-DI-BPM-035:Y", "SR-DI-BPM-036:Y", "SR-DI-BPM-037:Y", "SR-DI-BPM-041:Y", "SR-DI-BPM-042:Y", "SR-DI-BPM-043:Y", "SR-DI-BPM-044:Y", "SR-DI-BPM-045:Y", "SR-DI-BPM-046:Y", "SR-DI-BPM-047:Y", "SR-DI-BPM-048:Y", "SR-DI-BPM-050:Y", "SR-DI-BPM-051:Y", "SR-DI-BPM-052:Y", "SR-DI-BPM-053:Y", "SR-DI-BPM-054:Y", "SR-DI-BPM-055:Y", "SR-DI-BPM-056:Y", "SR-DI-BPM-057:Y", "SR-DI-BPM-061:Y", "SR-DI-BPM-062:Y", "SR-DI-BPM-063:Y", "SR-DI-BPM-064:Y", "SR-DI-BPM-065:Y", "SR-DI-BPM-066:Y", "SR-DI-BPM-067:Y", "SR-DI-BPM-071:Y", "SR-DI-BPM-072:Y", "SR-DI-BPM-073:Y", "SR-DI-BPM-074:Y", "SR-DI-BPM-075:Y", "SR-DI-BPM-076:Y", "SR-DI-BPM-077:Y", "SR-DI-BPM-081:Y", "SR-DI-BPM-082:Y", "SR-DI-BPM-083:Y", "SR-DI-BPM-084:Y", "SR-DI-BPM-085:Y", "SR-DI-BPM-086:Y", "SR-DI-BPM-087:Y", "SR-DI-BPM-091:Y", "SR-DI-BPM-092:Y", "SR-DI-BPM-093:Y", "SR-DI-BPM-094:Y", "SR-DI-BPM-095:Y", "SR-DI-BPM-096:Y", "SR-DI-BPM-097:Y", "SR-DI-BPM-101:Y", "SR-DI-BPM-102:Y", "SR-DI-BPM-103:Y", "SR-DI-BPM-104:Y", "SR-DI-BPM-105:Y", "SR-DI-BPM-106:Y", "SR-DI-BPM-107:Y", "SR-DI-BPM-111:Y", "SR-DI-BPM-112:Y", "SR-DI-BPM-113:Y", "SR-DI-BPM-114:Y", "SR-DI-BPM-115:Y", "SR-DI-BPM-116:Y", "SR-DI-BPM-117:Y", "SR-DI-BPM-121:Y", "SR-DI-BPM-122:Y", "SR-DI-BPM-123:Y", "SR-DI-BPM-124:Y", "SR-DI-BPM-125:Y", "SR-DI-BPM-126:Y", "SR-DI-BPM-127:Y", "SR-DI-BPM-128:Y", "SR-DI-BPM-130:Y", "SR-DI-BPM-131:Y", "SR-DI-BPM-132:Y", "SR-DI-BPM-133:Y", "SR-DI-BPM-134:Y", "SR-DI-BPM-135:Y", "SR-DI-BPM-136:Y", "SR-DI-BPM-137:Y", "SR-DI-BPM-141:Y", "SR-DI-BPM-142:Y", "SR-DI-BPM-143:Y", "SR-DI-BPM-144:Y", "SR-DI-BPM-145:Y", "SR-DI-BPM-146:Y", "SR-DI-BPM-147:Y", "SR-DI-BPM-151:Y", "SR-DI-BPM-152:Y", "SR-DI-BPM-153:Y", "SR-DI-BPM-154:Y", "SR-DI-BPM-155:Y", "SR-DI-BPM-156:Y", "SR-DI-BPM-157:Y", "SR-DI-BPM-161:Y", "SR-DI-BPM-162:Y", "SR-DI-BPM-163:Y", "SR-DI-BPM-164:Y", "SR-DI-BPM-165:Y", "SR-DI-BPM-166:Y", "SR-DI-BPM-167:Y", "SR-DI-BPM-171:Y", "SR-DI-BPM-172:Y", "SR-DI-BPM-173:Y", "SR-DI-BPM-174:Y", "SR-DI-BPM-175:Y", "SR-DI-BPM-176:Y", "SR-DI-BPM-177:Y", "SR-DI-BPM-181:Y", "SR-DI-BPM-182:Y", "SR-DI-BPM-183:Y", "SR-DI-BPM-184:Y", "SR-DI-BPM-185:Y", "SR-DI-BPM-186:Y", "SR-DI-BPM-187:Y", "SR-DI-BPM-191:Y", "SR-DI-BPM-192:Y", "SR-DI-BPM-193:Y", "SR-DI-BPM-194:Y", "SR-DI-BPM-195:Y", "SR-DI-BPM-196:Y", "SR-DI-BPM-197:Y", "SR-DI-BPM-201:Y", "SR-DI-BPM-202:Y", "SR-DI-BPM-203:Y", "SR-DI-BPM-204:Y", "SR-DI-BPM-205:Y", "SR-DI-BPM-206:Y", "SR-DI-BPM-207:Y", "SR-DI-BPM-208:Y", "SR-DI-BPM-210:Y", "SR-DI-BPM-211:Y", "SR-DI-BPM-212:Y", "SR-DI-BPM-213:Y", "SR-DI-BPM-214:Y", "SR-DI-BPM-215:Y", "SR-DI-BPM-216:Y", "SR-DI-BPM-217:Y", "SR-DI-BPM-221:Y", "SR-DI-BPM-222:Y", "SR-DI-BPM-223:Y", "SR-DI-BPM-224:Y", "SR-DI-BPM-225:Y", "SR-DI-BPM-226:Y", "SR-DI-BPM-227:Y", "SR-DI-BPM-231:Y", "SR-DI-BPM-232:Y", "SR-DI-BPM-233:Y", "SR-DI-BPM-234:Y", "SR-DI-BPM-235:Y", "SR-DI-BPM-236:Y", "SR-DI-BPM-237:Y", "SR-DI-BPM-241:Y", "SR-DI-BPM-242:Y", "SR-DI-BPM-243:Y", "SR-DI-BPM-244:Y", "SR-DI-BPM-245:Y", "SR-DI-BPM-246:Y", "SR-DI-BPM-247:Y"]  # sorted BPMY_174
    w136 = string[] ["SR-DI-BPM-011:X", "SR-DI-BPM-012:X", "SR-DI-BPM-013:X", "SR-DI-BPM-014:X", "SR-DI-BPM-015:X", "SR-DI-BPM-016:X", "SR-DI-BPM-017:X", "SR-DI-BPM-021:X", "SR-DI-BPM-022:X", "SR-DI-BPM-023:X", "SR-DI-BPM-024:X", "SR-DI-BPM-025:X", "SR-DI-BPM-026:X", "SR-DI-BPM-027:X", "SR-DI-BPM-031:X", "SR-DI-BPM-032:X", "SR-DI-BPM-033:X", "SR-DI-BPM-034:X", "SR-DI-BPM-035:X", "SR-DI-BPM-036:X", "SR-DI-BPM-037:X", "SR-DI-BPM-041:X", "SR-DI-BPM-042:X", "SR-DI-BPM-043:X", "SR-DI-BPM-044:X", "SR-DI-BPM-045:X", "SR-DI-BPM-046:X", "SR-DI-BPM-047:X", "SR-DI-BPM-048:X", "SR-DI-BPM-050:X", "SR-DI-BPM-051:X", "SR-DI-BPM-052:X", "SR-DI-BPM-053:X", "SR-DI-BPM-054:X", "SR-DI-BPM-055:X", "SR-DI-BPM-056:X", "SR-DI-BPM-057:X", "SR-DI-BPM-061:X", "SR-DI-BPM-062:X", "SR-DI-BPM-063:X", "SR-DI-BPM-064:X", "SR-DI-BPM-065:X", "SR-DI-BPM-066:X", "SR-DI-BPM-067:X", "SR-DI-BPM-071:X", "SR-DI-BPM-072:X", "SR-DI-BPM-073:X", "SR-DI-BPM-074:X", "SR-DI-BPM-075:X", "SR-DI-BPM-076:X", "SR-DI-BPM-077:X", "SR-DI-BPM-081:X", "SR-DI-BPM-082:X", "SR-DI-BPM-083:X", "SR-DI-BPM-084:X", "SR-DI-BPM-085:X", "SR-DI-BPM-086:X", "SR-DI-BPM-087:X", "SR-DI-BPM-091:X", "SR-DI-BPM-092:X", "SR-DI-BPM-093:X", "SR-DI-BPM-094:X", "SR-DI-BPM-095:X", "SR-DI-BPM-096:X", "SR-DI-BPM-097:X", "SR-DI-BPM-101:X", "SR-DI-BPM-102:X", "SR-DI-BPM-103:X", "SR-DI-BPM-104:X", "SR-DI-BPM-105:X", "SR-DI-BPM-106:X", "SR-DI-BPM-107:X", "SR-DI-BPM-111:X", "SR-DI-BPM-112:X", "SR-DI-BPM-113:X", "SR-DI-BPM-114:X", "SR-DI-BPM-115:X", "SR-DI-BPM-116:X", "SR-DI-BPM-117:X", "SR-DI-BPM-121:X", "SR-DI-BPM-122:X", "SR-DI-BPM-123:X", "SR-DI-BPM-124:X", "SR-DI-BPM-125:X", "SR-DI-BPM-126:X", "SR-DI-BPM-127:X", "SR-DI-BPM-128:X", "SR-DI-BPM-130:X", "SR-DI-BPM-131:X", "SR-DI-BPM-132:X", "SR-DI-BPM-133:X", "SR-DI-BPM-134:X", "SR-DI-BPM-135:X", "SR-DI-BPM-136:X", "SR-DI-BPM-137:X", "SR-DI-BPM-141:X", "SR-DI-BPM-142:X", "SR-DI-BPM-143:X", "SR-DI-BPM-144:X", "SR-DI-BPM-145:X", "SR-DI-BPM-146:X", "SR-DI-BPM-147:X", "SR-DI-BPM-151:X", "SR-DI-BPM-152:X", "SR-DI-BPM-153:X", "SR-DI-BPM-154:X", "SR-DI-BPM-155:X", "SR-DI-BPM-156:X", "SR-DI-BPM-157:X", "SR-DI-BPM-161:X", "SR-DI-BPM-162:X", "SR-DI-BPM-163:X", "SR-DI-BPM-164:X", "SR-DI-BPM-165:X", "SR-DI-BPM-166:X", "SR-DI-BPM-167:X", "SR-DI-BPM-171:X", "SR-DI-BPM-172:X", "SR-DI-BPM-173:X", "SR-DI-BPM-174:X", "SR-DI-BPM-175:X", "SR-DI-BPM-176:X", "SR-DI-BPM-177:X", "SR-DI-BPM-181:X", "SR-DI-BPM-182:X", "SR-DI-BPM-183:X", "SR-DI-BPM-184:X", "SR-DI-BPM-185:X", "SR-DI-BPM-186:X", "SR-DI-BPM-187:X", "SR-DI-BPM-191:X", "SR-DI-BPM-192:X", "SR-DI-BPM-193:X", "SR-DI-BPM-194:X", "SR-DI-BPM-195:X", "SR-DI-BPM-196:X", "SR-DI-BPM-197:X", "SR-DI-BPM-201:X", "SR-DI-BPM-202:X", "SR-DI-BPM-203:X", "SR-DI-BPM-204:X", "SR-DI-BPM-205:X", "SR-DI-BPM-206:X", "SR-DI-BPM-207:X", "SR-DI-BPM-208:X", "SR-DI-BPM-210:X", "SR-DI-BPM-211:X", "SR-DI-BPM-212:X", "SR-DI-BPM-213:X", "SR-DI-BPM-214:X", "SR-DI-BPM-215:X", "SR-DI-BPM-216:X", "SR-DI-BPM-217:X", "SR-DI-BPM-221:X", "SR-DI-BPM-222:X", "SR-DI-BPM-223:X", "SR-DI-BPM-224:X", "SR-DI-BPM-225:X", "SR-DI-BPM-226:X", "SR-DI-BPM-227:X", "SR-DI-BPM-231:X", "SR-DI-BPM-232:X", "SR-DI-BPM-233:X", "SR-DI-BPM-234:X", "SR-DI-BPM-235:X", "SR-DI-BPM-236:X", "SR-DI-BPM-237:X", "SR-DI-BPM-241:X", "SR-DI-BPM-242:X", "SR-DI-BPM-243:X", "SR-DI-BPM-244:X", "SR-DI-BPM-245:X", "SR-DI-BPM-246:X", "SR-DI-BPM-247:X"]  # sorted BPMX_174
    w199 = string[] ["BL-05A:HutchA_Enable", "BL-09A:HutchA_Enable", "BL-21A:HutchA_Enable", "BL-23A:HutchA_Enable", "BL-25A:HutchA_Enable", "BL-41A:HutchA_Enable", "BL-45A:HutchA_Enable"]  # Hutch enable
    w218 = string[] ["CPCI03-adl7452-0:doBank0Ch5", "CPCI05-adl7452-0:doBank0Ch5", "CPCI11-adl7452-0:doBank0Ch5", "CPCI12-adl7452-0:doBank0Ch5", "CPCI13-adl7452-0:doBank0Ch5", "CPCI21-adl7452-0:doBank0Ch5", "CPCI23-adl7452-0:doBank0Ch5"]  # FE enable
    (unwired) 1 ("index")
    w295 = 578.303 ("y")
    w300 = 1.202 ("y")
    # "FE-DI-XBPM-051:SA:SA_Y_MONITOR"
    # "FE-DI-XBPM-051:SA:SA_X_MONITOR"
    # "0為"
    # "05\n09\n21\n23\n25\n41\n45"
    # "gapMotorOff"
    n2 = disable-structure shown="Disabled" {
      frame Disabled {
        n3 = call-poly <userlib>:"CaLabGet.vi"("PV Name"="TI-INJ-PROC:getTrig-LI-EGUN") -> ("1rst Value (string)"=w324:string)  [unwired: 8 in, 6 out]
        n4 = Equal?(x="1" ("1rst Value (string)"), y=w324) -> (x = y?=w322:bool)
        n5 = case shown="True" w322 {
          frame False {
          }
          frame True {
            n6 = local read item#-1() -> (→"date (last Gun ON)")
            n7 = local read item#-1() -> (→"time string (last Gun ON)")
          }
        }
      }
      frame Enabled {
      }
    }
    n8 = disable-structure shown="Disabled" {
      frame Disabled {
        n9 = To Long Integer() -> (32bit integer=w364:i32)  [unwired: 1 in]
        n10 = case shown="1" w364 {
          tunnel: ["Decay" "Top-Up"] -> _
          frame 0, Default {
          }
          frame 1 {
          }
        }
      }
      frame Enabled {
      }
    }
    n11 = call-poly <userlib>:"CaLabGet.vi"("PV Names"=string[] ["LI-ES-CPS-01:PULSEMODE", "LI-ES-BPS-01:SETU:GRID", "LI-ES-BPS-01:SETU:MBM", "LI-ES-BPS-01:SETU:SBM", "LI-RF-HVP-31:SET:U", "CPCITM-TI-EVRTG:Pulse6DelaySet", "CPCITM-TI-EVRTG:Pulse7DelaySet", "CPCITM-TI-EVRTG:Pulse6WidthSet", "CPCITM-TI-EVRTG:Pulse7WidthSet", "CPCITM-TI-EVRTG:GTX6CtrlGTXPHSet", "CPCITM-TI-EVRTG:GTX7CtrlGTXPHSet", "CPCITM-TI-EVRTG:GTX6DlySet", "CPCITM-TI-EVRTG:GTX7DlySet"]) -> ("1rst Value (string)"=w228:string[], "1rst Value (number)"=w279:dbl[])  [unwired: 8 in, 5 out]
    "Value Array (number) 3" <- w279
    "1rst Value (string) 2" <- w228
    n12 = call-poly <userlib>:"CaLabGet.vi"("PV Names"=string[] ["BR-PS-INJ-SE:setHV", "BR-PS-INJ-KI:setHV", "BR-PS-EXT-K1:setHV", "BR-PS-EXT-K2:setHV", "BR-PS-EXT-SE1:setHV", "BR-PS-EXT-SE2:setHV", "SR-PS-INJ-SE1:setHV", "SR-PS-INJ-SE2:setHV", "SR-PS-INJ-K1:setHV", "SR-PS-INJ-K2:setHV", "SR-PS-INJ-K3:setHV", "SR-PS-INJ-K4:setHV"]) -> ("1rst Value (number)"=w281:dbl[])  [unwired: 8 in, 6 out]
    "Value Array (number) 2" <- w281
    n13 = call-poly <userlib>:"CaLabGet.vi"("PV Names"=string[] ["SR-RF-MSG:setFreq", "SR-RF2-LLRF:local", "SR-RF2-LLRF:getOperationMode", "SR-RF2-LLRF:getGapVoltage", "SR-RF2-LLRF:setGapVoltage", "SR-RF2-LLRF:setStationPhase", "SR-RF3-LLRF:local", "SR-RF3-LLRF:getOperationMode", "SR-RF3-LLRF:getGapVoltage", "SR-RF3-LLRF:setGapVoltage", "SR-RF3-LLRF:setStationPhase"]) -> ("1rst Value (number)"=w254:dbl[])  [unwired: 8 in, 6 out]
    "Value Array (number) 4" <- w254
    n14 = call-poly <userlib>:"CaLabGet.vi"("PV Names"=string[] ["SR-DI-FP:CurrentBuffer"]) -> ("Value Array (number)"=w236:dbl[][])  [unwired: 8 in, 6 out]
    n15 = call-poly <userlib>:"CaLabGet.vi"("PV Names"=string[] ["TI-INJ-PROC:TopupHiLowStart", "SR-DI-DCCT:BeamCurrent", "SR-DI-DCCT:BeamLifetime", "SR-DI-XPC-40:SigmaX", "SR-DI-XPC-40:SigmaY", "SR-DI-TUNE:nux", "SR-DI-TUNE:nuy", "IGPF:TPSX:SRAM:VEC:PEAKFREQ2", "IGPF:TPSY:SRAM:VEC:PEAKFREQ2", "TI-INJ-PROC:setBucketAddressStart", "TI-INJ-PROC:setBucketAddressLast", "TI-INJ-PROC:setBucketAddressStep"]) -> ("1rst Value (number)"=w315:dbl[])  [unwired: 8 in, 6 out]
    "Value Array (number)" <- w315
    n16 = call-poly <userlib>:"CaLabGet.vi"("PV Names"=string[] ["LI:restoreFilename", "LTB:restoreFilename", "BR:restoreFilename", "BTS:restoreFilename", "SR:restoreFilename"]) -> ("1rst Value (string)"=w238:string[])  [unwired: 8 in, 6 out]
    "1rst Value (string)" <- w238
    n17 = Index Array(array=w228, index=0) -> (element=w226:string)
    n18 = Index Array(array=w279, index #1=0 ("index"), index #2=1 ("index"), index #3=2 ("index"), index #4=3 ("index"), index #5=4 ("index"), index #6=5 ("index"), index #7=6 ("index"), index #8=7 ("index"), index #9=8 ("index"), index #10=9 ("index"), index #11=10 ("index"), index #12=11 ("index"), index #13=12 ("index")) -> (element #2=w110:dbl, element #3=w230:dbl, element #4=w229:dbl, element #5=w108:dbl, element #8=w225:dbl, element #9=w224:dbl, element #10=w223:dbl, element #11=w222:dbl, element #12=w221:dbl, element #13=w220:dbl)  [unwired: 3 out]
    "MBM volt.(S)" <- w230
    "SBM volt.(S)" <- w229
    n19 = Index Array(array=w281, index #1=0 ("index"), index #2=1 ("index"), index #3=2 ("index"), index #4=3 ("index"), index #5=4 ("index"), index #6=5 ("index"), index #7=6 ("index"), index #8=7 ("index"), index #9=8 ("index"), index #10=9 ("index"), index #11=10 ("index"), index #12=11 ("index")) -> (element #1=w123:dbl, element #2=w122:dbl, element #3=w121:dbl, element #4=w120:dbl, element #5=w119:dbl, element #6=w118:dbl, element #7=w117:dbl, element #8=w116:dbl, element #9=w115:dbl, element #10=w114:dbl, element #11=w113:dbl, element #12=w112:dbl)
    n20 = Index Array(array=w254, index #1=0 ("index"), index #2=1 ("index"), index #3=2 ("index"), index #4=3 ("index"), index #5=4 ("index"), index #6=5 ("index"), index #7=6 ("index"), index #8=7 ("index"), index #9=8 ("index"), index #10=9 ("index"), index #11=10 ("index")) -> (element #1=w102:dbl, element #2=w251:dbl, element #3=w249:dbl, element #5=w8:dbl, element #6=w9:dbl, element #7=w246:dbl, element #8=w245:dbl, element #10=w98:dbl, element #11=w99:dbl)  [unwired: 2 out]
    n21 = Index Array(array=w236, index (row)=0 ("index")) -> (element=w92:dbl[])  [unwired: 1 in]
    n22 = Index Array(array=w315, index #1=0 ("index"), index #2=1 ("index"), index #3=2 ("index"), index #4=3 ("index"), index #5=4 ("index"), index #6=5 ("index"), index #7=6 ("index"), index #8=7 ("index"), index #9=8 ("index"), index #10=9 ("index"), index #11=10 ("index"), index #12=11 ("index")) -> (element #1=w313:dbl, element #2=w132:dbl, element #3=w131:dbl, element #4=w301:dbl, element #5=w299:dbl, element #6=w298:dbl, element #7=w297:dbl, element #8=w296:dbl, element #9=w294:dbl, element #10=w126:dbl, element #11=w125:dbl, element #12=w124:dbl)
    n23 = Index Array(array=w238, index #1=0 ("index"), index #2=1 ("index"), index #3=2 ("index"), index #4=3 ("index"), index #5=4 ("index")) -> (element #1=w94:string, element #2=w93:string, element #3=w97:string, element #4=w96:string, element #5=w95:string)
    n24 = call-poly <userlib>:"CaLabGet.vi"("PV Names"=w199) -> ("1rst Value (string)"=w207:string[])  [unwired: 8 in, 6 out]
    n25 = for {
      tunnel: w207 -> [w333] mode=indexing
      tunnel: [w332] -> w208 mode=indexing
      n26 = case shown="\"Enable\"" w333 {
        tunnel: [FALSE TRUE] -> w332
        frame "Disable", Default {
        }
        frame "Enable" {
        }
      }
    }
    n27 = call-poly <userlib>:"CaLabGet.vi"("PV Names"=w218) -> ("1rst Value (string)"=w210:string[])  [unwired: 8 in, 6 out]
    n28 = call-poly <userlib>:"CaLabGet.vi"("PV Names"=string[] ["SR-ID-IU22-05:getGap", "SR-ID-IU22A-09:getGap", "SR-ID-IU22B-09:getGap", "SR-ID-IUT22-21:getGap", "SR-ID-IU22-23:getGap", "SR-ID-IU22A-25:getGap", "SR-ID-IU22B-25:getGap", "SR-ID-EPU48A-41:getGap", "SR-ID-EPU48A-41:getPhase", "SR-ID-EPU48B-41:getGap", "SR-ID-EPU48B-41:getPhase", "SR-ID-EPU46-45:getGap", "SR-ID-EPU46-45:getPhase", "SR-ID-IUT22-21:getGapTaper", "SR-ID-EPU48PS-41:getGap"]) -> ("1rst Value (number)"=w198:dbl[])  [unwired: 8 in, 6 out]
    "Value Array (number) 6" <- w198
    n29 = for {
      tunnel: w210 -> [w337] mode=indexing
      tunnel: [w336] -> w209 mode=indexing
      n30 = case shown="\"disable\", Default" w337 {
        tunnel: [FALSE TRUE] -> w336
        frame "disable", Default {
        }
        frame "enable" {
        }
      }
    }
    n31 = call-poly <userlib>:"CaLabGet.vi"("PV Names"=string[] ["SR-ID-IU22-05:gapMotorOff", "SR-ID-IU22A-09:gapMotorOff", "SR-ID-IU22B-09:gapMotorOff", "SR-ID-IUT22-21:gapMotorOff", "SR-ID-IU22-23:gapMotorOff", "SR-ID-IU22A-25:gapMotorOff", "SR-ID-IU22B-25:gapMotorOff", "SR-ID-EPU48A-41:gapMotorOff", "SR-ID-EPU48B-41:gapMotorOff", "SR-ID-EPU46-45:gapMotorOff", "SR-ID-EPU48A-41:phaseMotorOff", "SR-ID-EPU48B-41:phaseMotorOff", "SR-ID-EPU46-45:phaseMotorOff"]) -> ("1rst Value (string)"=w149:string[])  [unwired: 8 in, 6 out]
    n32 = To Long Integer(number=w249) -> (32bit integer=w250:i32)
    n33 = To Long Integer(number=w251) -> (32bit integer=w252:i32)
    n34 = To Long Integer(number=w245) -> (32bit integer=w248:i32)
    n35 = call-poly <userlib>:"CaLabGet.vi"("PV Names"=string[] ["FE-DI-XBPM-051:signals:sa.X", "FE-DI-XBPM-051:signals:sa.Y", "FE-DI-XBPM-091:SA:SA_X_MONITOR", "FE-DI-XBPM-091:SA:SA_Y_MONITOR", "FE-DI-XBPM-211:SA:SA_X_MONITOR", "FE-DI-XBPM-211:SA:SA_Y_MONITOR", "FE-DI-XBPM-231:SA:SA_X_MONITOR", "FE-DI-XBPM-231:SA:SA_Y_MONITOR", "FE-DI-XBPM-251:SA:SA_X_MONITOR", "FE-DI-XBPM-251:SA:SA_Y_MONITOR", "FE-DI-XBPM-411:SA:SA_X_MONITOR", "FE-DI-XBPM-411:SA:SA_Y_MONITOR", "FE-DI-XBPM-451:SA:SA_X_MONITOR", "FE-DI-XBPM-451:SA:SA_Y_MONITOR"]) -> ("1rst Value (number)"=w165:dbl[])  [unwired: 8 in, 6 out]
    n36 = To Long Integer(number=w246) -> (32bit integer=w247:i32)
    n37 = Index Array(array=w198, index #1=0 ("index"), index #2=1 ("index"), index #3=2 ("index"), index #4=3 ("index"), index #5=4 ("index"), index #6=5 ("index"), index #7=6 ("index"), index #8=7 ("index"), index #9=8 ("index"), index #10=9 ("index"), index #11=10 ("index"), index #12=11 ("index"), index #13=12 ("index"), index #14=13 ("index"), index #15=14 ("index")) -> (element #1=w76:dbl, element #2=w75:dbl, element #3=w74:dbl, element #4=w73:dbl, element #5=w72:dbl, element #6=w71:dbl, element #7=w70:dbl, element #8=w69:dbl, element #9=w68:dbl, element #10=w67:dbl, element #11=w66:dbl, element #12=w65:dbl, element #13=w64:dbl, element #14=w7:dbl, element #15=w63:dbl)
    n38 = for {
      tunnel: w149 -> [w329] mode=indexing
      tunnel: [w328] -> w148 mode=indexing
      n39 = case shown="\"0\"" w329 {
        tunnel: [FALSE TRUE] -> w328
        frame "1", Default {
        }
        frame "0" {
        }
      }
    }
    n40 = case shown="0, Default" w252 {
      tunnel: [FALSE TRUE] -> w104
      frame 0, Default {
      }
      frame 1 {
      }
    }
    n41 = case shown="0, Default" w247 {
      tunnel: [FALSE TRUE] -> w101
      frame 0, Default {
      }
      frame 1 {
      }
    }
    n42 = case shown="0" w250 {
      tunnel: [TRUE FALSE] -> w103
      frame 0 {
      }
      frame 1, Default {
      }
    }
    n43 = case shown="0" w248 {
      tunnel: [TRUE FALSE] -> w100
      frame 0 {
      }
      frame 1, Default {
      }
    }
    n44 = Multiply(x=w165, y=0.001) -> (x*y=w164:dbl[])
    "Value Array (number) 7" <- w164
    n45 = To Long Integer(number=w313) -> (32bit integer=w316:i32)
    n46 = Negate(x=w7) -> (-x=w6:dbl)
    n47 = Index Array(array=w164, index #1=0 ("index"), index #2=1 ("index"), index #3=2 ("index"), index #4=3 ("index"), index #5=4 ("index"), index #6=5 ("index"), index #7=6 ("index"), index #8=7 ("index"), index #9=8 ("index"), index #10=9 ("index"), index #11=10 ("index"), index #12=11 ("index"), index #13=12 ("index"), index #14=13 ("index")) -> (element #1=w62:dbl, element #2=w55:dbl, element #3=w61:dbl, element #4=w54:dbl, element #5=w60:dbl, element #6=w53:dbl, element #7=w59:dbl, element #8=w52:dbl, element #9=w58:dbl, element #10=w51:dbl, element #11=w57:dbl, element #12=w50:dbl, element #13=w56:dbl, element #14=w49:dbl)
    n48 = case shown="1" w316 {
      tunnel: ["Decay" "Top-Up"] -> w133
      frame 0, Default {
      }
      frame 1 {
      }
    }
    n49 = Index Array(array=w208, index #1=0 ("index"), index #2=1 ("index"), index #3=2 ("index"), index #4=3 ("index"), index #5=4 ("index"), index #6=5 ("index"), index #7=6 ("index")) -> (element #1=w83:bool, element #2=w82:bool, element #3=w81:bool, element #4=w80:bool, element #5=w79:bool, element #6=w78:bool, element #7=w77:bool)
    n50 = case shown="\"MBM\", Default" w226 {
      tunnel: ["MBM" "SBM"] -> w111
      tunnel: w230 -> [w343 _]
      tunnel: [w343 w348] -> w109
      tunnel: w229 -> [_ w348]
      tunnel: w225 -> [_ w347]
      tunnel: w224 -> [w342 _]
      tunnel: [w342 w347] -> w107
      tunnel: w223 -> [_ w346]
      tunnel: w222 -> [w341 _]
      tunnel: [w341 w346] -> w106
      tunnel: w221 -> [_ w345]
      tunnel: w220 -> [w340 _]
      tunnel: [w340 w345] -> w105
      frame "MBM", Default {
      }
      frame "SBM" {
      }
    }
    n51 = Multiply(x=w301, y=w300) -> (x*y=w130:dbl)
    n52 = Divide(x=w296, y=w295) -> (x/y=w128:dbl)
    n53 = Multiply(x=w299, y=w300) -> (x*y=w129:dbl)
    n54 = Divide(x=w294, y=w295) -> (x/y=w127:dbl)
    n55 = Index Array(array=w209, index #1=0 ("index"), index #2=1 ("index"), index #3=2 ("index"), index #4=3 ("index"), index #5=4 ("index"), index #6=5 ("index"), index #7=6 ("index")) -> (element #1=w90:bool, element #2=w89:bool, element #3=w88:bool, element #4=w87:bool, element #5=w86:bool, element #6=w85:bool, element #7=w84:bool)
    n56 = call-poly <userlib>:"CaLabGet.vi"("PV Name"="TI-INJ-PROC:getTrig-SR-KICKER") -> ("1rst Value (string)"=w233:string)  [unwired: 8 in, 6 out]
    n57 = Index Array(array=w148, index #1=0 ("index"), index #2=1 ("index"), index #3=2 ("index"), index #4=3 ("index"), index #5=4 ("index"), index #6=5 ("index"), index #7=6 ("index"), index #8=7 ("index"), index #9=8 ("index"), index #10=9 ("index"), index #11=10 ("index"), index #12=11 ("index"), index #13=12 ("index")) -> (element #1=w48:bool, element #2=w47:bool, element #3=w46:bool, element #4=w45:bool, element #5=w44:bool, element #6=w43:bool, element #7=w42:bool, element #8=w41:bool, element #9=w40:bool, element #10=w39:bool, element #11=w38:bool, element #12=w37:bool, element #13=w36:bool)
    n58 = Equal?(x="1" ("1rst Value (string)"), y=w233) -> (x = y?=w231:bool)
    "x = y?" <- w231
    n59 = call-poly <userlib>:"CaLabGet.vi"("PV Names"=string[] ["SR-DI-FOFB-H:getStatus", "SR-DI-FOFB-V:getStatus", "IGPF:TPSX:FBCTRL", "IGPF:TPSY:FBCTRL", "TPS-SR-022:bpm4:ilk:enabled", "SR-DI-ANGLE-ILK:StatusX", "SR-DI-ANGLE-ILK:StatusY"]) -> ("1rst Value (string)"=w22:string[], "1rst Value (number)"=w23:dbl[])  [unwired: 8 in, 5 out]
    n60 = call-poly <userlib>:"CaLabGet.vi"("PV Names"=w136) -> ("1rst Value (number)"=w138:dbl[])  [unwired: 8 in, 6 out]
    n61 = call-poly <userlib>:"CaLabGet.vi"("PV Names"=w137) -> ("1rst Value (number)"=w141:dbl[])  [unwired: 8 in, 6 out]
    n62 = To Byte Integer(number=w23) -> (8bit integer=w19:i8[])
    n63 = for {
      tunnel: w19 -> [w319] mode=indexing
      tunnel: [w318] -> w29 mode=indexing
      n64 = case shown="1" w319 {
        tunnel: [TRUE FALSE] -> w318
        frame 1 {
        }
        frame 0, Default {
        }
      }
    }
    n65 = Multiply(x=w138, y=w140) -> (x*y=w139:dbl[])
    n66 = Multiply(x=w141, y=w140) -> (x*y=w142:dbl[])
    n67 = case shown="True" w231 {
      tunnel: w298 -> [_ w353]
      tunnel: w297 -> [_ w352]
      tunnel: [w351 w353] -> w5
      tunnel: [w350 w352] -> w4
      tunnel: w3 -> [w351 _]
      tunnel: w2 -> [w350 _]
      frame False {
      }
      frame True {
        n68 = local read "NOW date"() -> (→"date kickeron":string)
        n69 = local read "NOW time"() -> (→"time kickeron":string)
      }
    }
    n70 = Index Array(array=w22, index #1=0 ("index"), index #2=1 ("index")) -> (element #1=w17:string, element #2=w16:string)
    n71 = Wait Until Next ms Multiple(millisecond multiple=u32 1000) -> ()  [unwired: 1 out]
    n72 = local read "date kickeron"() -> (w11:string)
    n73 = local read "time kickeron"() -> (w10:string)
    n74 = Index Array(array=w29, index #1=2 ("index"), index #2=3 ("index"), index #3=4 ("index"), index #4=5 ("index"), index #5=6 ("index")) -> (element #1=w15:bool, element #2=w14:bool, element #3=w13:bool)  [unwired: 2 out]
    n75 = Bundle("Array 4"=w143, w139) -> (w35:cluster{"Array 4":i32[], dbl[]})  [unwired: 1 in]
    n76 = Bundle("Array 4"=w143, w142) -> (w34:cluster{"Array 4":i32[], dbl[]})  [unwired: 1 in]
    n77 = Get Date/Time In Seconds() -> (seconds since 1Jan1904=w145:timestamp)
    n78 = Format Date/Time String(time format string (%c)="%Y\\%m\\%d", seconds (now)=w145) -> (date/time string=→"NOW date":string)  [unwired: 1 in]
    n79 = Format Date/Time String(time format string (%c)="%Y/%m/%d", seconds (now)=w145) -> (date/time string=w33:string)  [unwired: 1 in]
    n80 = Format Date/Time String(time format string (%c)="%H:%M:%S", seconds (now)=w145) -> (date/time string=w32:string)  [unwired: 1 in]
    "NOW time" <- w32
    n81 = Bundle By Name(cluster=T2 {"SR Fill Pattern"=array[10000 elements], "Beam Current(mA"=302.073574, "Beam Lifetime(min)"=665.9266107283645, "Beamsize X(um)"=55.88912339231618, "Beamsize Y(um)"=33.47785442299371, "Tune X(form BPM)"=0.14677103718199608, "Tune Y(form BPM)"=0.2162426614481409, "Mode"="Top-Up", "NuX(form BBF) "=0.1781877868128751, "NuY(form BBF)"=0.25219386232318686, "IU22-23gap(R)"=11.0, "IU22-05gap(R)"=7.29, "IU22-05M"=FALSE, "IU22A-09gap(R)"=8.074, "IU22A-09M"=FALSE, "IU22B-09gap(R)"=40.001, "IU22B-09M"=FALSE, "IUT22-21gap(R)"=7.0, "IUT22-21M"=FALSE, "IU22-23M"=FALSE, "IU22A-25gap(R)"=8.18, "IU22A-25M"=FALSE, "IU22B-25gap(R)"=40.0, "IU22B-25M"=FALSE, "EPU48A-41gap(R)"=64.99985000000001, "EPU48A-41gM"=FALSE, "EPU48B-41gap(R)"=65.00399999999999, "EPU48B-41gM"=FALSE, "EPU46-45gap(R)"=44.9999, "EPU46-45gM"=FALSE, "EPU48A-41phase(R)"=0.0001, "EPU48B-41phase(R)"=0.00055, "EPU46-45phase(R)"=0.00025, "Grid volt.(S)"=33.0, "Gun mode"="MBM", "Mod.3 HV(S)"=35.800000000000026, "SR"="Booster_JT_2016_1005_1200.data", "BR"="BTS_2016_1116_1020.data", "Linac"="Linac2016_1005_0935.data", "LTB"="LTB_JT_2016_1005_1200.data", "BTS"="SR_DMB_2016_1102_1124LOCO.data", "RF2 remote"=TRUE, "RF2 OP mode"=TRUE, "RF2 phase.(S)"=-56.70000000000001, "RF Freq.(s)"=499654659.7918481, "RF2 gap volt.(S)"=1400.0, "RF3 remote"=TRUE, "RF3 OP mode"=TRUE, "RF3 phase.(S)"=160.0, "RF3 gap volt.(S)"=1400.0, "BBF V"=FALSE, "BBF H"=FALSE, "BR ext. kicker1"=18.266, "BR ext. kicker2"=18.26600000000001, "BR ext. sep.1"=318.8444, "BR ext. sep.2"=444.5, "BR inj. sep."=105.2, "BR inj. kicker"=16.40000000000001, "SR kicker4"=8.27, "SR kicker3"=8.315, "SR kicker2"=8.325, "SR kicker1"=8.4, "SR inj. sep.2"=417.0, "SR inj. sep.1"=419.3416, "Bucket Start"=100.0, "Bucket Last"=630.0, "Bucket Step"=10.0, "Orbit ILK(P)"=FALSE, "IU22-05 Hutch Enable"=TRUE, "IU22A-09M Hutch Enable"=TRUE, "IUT22-21M Hutch Enable"=TRUE, "IU22-23M Hutch Enable"=FALSE, "IU22A-25M Hutch Enable"=TRUE, "EPU48A-41M Hutch Enable"=FALSE, "EPU46-45M Hutch Enable"=TRUE, "EPU46-45 FE Enable"=TRUE, "EPU48A-41 FE Enable"=FALSE, "IU22A-25 FE Enable"=TRUE, "IU22-23 FE Enable"=FALSE, "IUT22-21 FE Enable"=TRUE, "IU22A-09 FE Enable"=TRUE, "IU22-05 FE Enable"=TRUE, "EPU48A-41pM"=FALSE, "EPU48B-41pM"=FALSE, "EPU46-45pM"=FALSE, "Gun volt.(S)"=23.5, "Width count"=30.0, "2ns step"=0.0, "10ps delay"=100.0, "phase shifter"=130.00060000000002, "Taper"=-1.0899999999999999, "05XBPMX 1"=0.0, "09XBPMX 1"=0.0, "21XBPMX 1"=0.0, "23XBPMX 1"=0.0, "25XBPMX 1"=0.0, "41XBPMX 1"=0.0, "45XBPMX 1"=0.0, "05XBPMY 1"=0.0, "09XBPMY 1"=0.0, "21XBPMY 1"=0.0, "23XBPMY 1"=0.0, "25XBPMY 1"=0.0, "41XBPMY 1"=0.0, "45XBPMY 1"=0.0, "FOFB H"="MBM", "FOFB V"="MBM", "time string"="23:28:50", "date"="2016/08/29", "date (last kicker ON)"="2016/08/29", "time string (last kicker ON)"="23:28:50", "BPMX Graph"={[], "1rst Value (number)"=[]}, "BPMY Graph"={[], "1rst Value (number)"=[]}, "Radio Buttons 2"=enum."different with"} ("Cluster"), "Tune X(form BPM)"=w5, "Tune Y(form BPM)"=w4, "date (last kicker ON)"=w11, "time string (last kicker ON)"=w10, "date"=w33, "time string"=w32, "Mode"=w133, "Beam Current(mA"=w132, "Beam Lifetime(min)"=w131, "Beamsize X(um)"=w130, "Beamsize Y(um)"=w129, "NuX(form BBF)"=w128, "NuY(form BBF)"=w127, "Bucket Start"=w126, "Bucket Last"=w125, "Bucket Step"=w124, "BR inj. sep."=w123, "BR inj. kicker"=w122, "BR ext. kicker1"=w121, "BR ext. kicker2"=w120, "BR ext. sep.1"=w119, "BR ext. sep.2"=w118, "SR inj. sep.1"=w117, "SR inj. sep.2"=w116, "SR kicker1"=w115, "SR kicker2"=w114, "SR kicker3"=w113, "SR kicker4"=w112, "Gun mode"=w111, "Grid volt.(S)"=w110, "Gun volt.(S)"=w109, "Mod.3 HV(S)"=w108, "Width count"=w107, "2ns step"=w106, "10ps delay"=w105, "RF2 remote"=w104, "RF2 OP mode"=w103, "RF2 phase.(S)"=w9, "RF Freq.(s)"=w102, "RF2 gap volt.(S)"=w8, "RF3 remote"=w101, "RF3 OP mode"=w100, "RF3 phase.(S)"=w99, "RF3 gap volt.(S)"=w98, "BR"=w97, "BTS"=w96, "Linac"=w94, "LTB"=w93, "SR"=w95, "SR Fill Pattern"=w92, "IU22-05 Hutch Enable"=w83, "IU22A-09M Hutch Enable"=w82, "IUT22-21M Hutch Enable"=w81, "IU22-23M Hutch Enable"=w80, "IU22A-25M Hutch Enable"=w79, "EPU48A-41M Hutch Enable"=w78, "EPU46-45M Hutch Enable"=w77, "EPU46-45 FE Enable"=w84, "EPU48A-41 FE Enable"=w85, "IU22A-25 FE Enable"=w86, "IU22-23 FE Enable"=w87, "IUT22-21 FE Enable"=w88, "IU22A-09 FE Enable"=w89, "IU22-05 FE Enable"=w90, "IU22-05gap(R)"=w76, "IU22A-09gap(R)"=w75, "IU22B-09gap(R)"=w74, "IUT22-21gap(R)"=w73, "IU22-23gap(R)"=w72, "IU22A-25gap(R)"=w71, "IU22B-25gap(R)"=w70, "EPU48A-41gap(R)"=w69, "EPU48A-41phase(R)"=w68, "EPU48B-41gap(R)"=w67, "EPU48B-41phase(R)"=w66, "EPU46-45gap(R)"=w65, "EPU46-45phase(R)"=w64, "Taper"=w6, "phase shifter"=w63, "05XBPMX 1"=w62, "09XBPMX 1"=w61, "21XBPMX 1"=w60, "23XBPMX 1"=w59, "25XBPMX 1"=w58, "41XBPMX 1"=w57, "45XBPMX 1"=w56, "05XBPMY 1"=w55, "09XBPMY 1"=w54, "21XBPMY 1"=w53, "23XBPMY 1"=w52, "25XBPMY 1"=w51, "41XBPMY 1"=w50, "45XBPMY 1"=w49, "IU22-05M"=w48, "IU22A-09M"=w47, "IU22B-09M"=w46, "IUT22-21M"=w45, "IU22-23M"=w44, "IU22A-25M"=w43, "IU22B-25M"=w42, "EPU48A-41gM"=w41, "EPU48B-41gM"=w40, "EPU46-45gM"=w39, "EPU48A-41pM"=w38, "EPU48B-41pM"=w37, "EPU46-45pM"=w36, "BPMX Graph"=w35, "BPMY Graph"=w34, "Radio Buttons 2"=enum32{"absolute", "different with"}."absolute", "FOFB H"=w17, "FOFB V"=w16, "BBF H"=w15, "BBF V"=w14, "Orbit ILK(P)"=w13) -> (→"Cluster":T2)
  }
  n82 = while {
    i -> [w371]
    stop <- w369 stop-if-true
    # "D:\\LOG運轉紀錄\\2016"
    n83 = event shown="[2] \"Open Button\": Value Change" {
      selector: _ -> [_ _ _ _]
      dyn-events: _ -> [_ _ _ _]
      timeout: 233 -> [_ _ _ _]
      tunnel: [_ TRUE ("stop") _ _] -> w373
      event Timeout {
        n84 = event-data() -> ()  [unwired: 1 in, 3 out]
      }
      event "stop": Value Change {
        n85 = event-data() -> ()  [unwired: 1 in, 4 out]
      }
      event "Open Button": Value Change {
        n86 = event-data() -> ()  [unwired: 1 in, 6 out]
        n87 = Get Date/Time In Seconds() -> (seconds since 1Jan1904=w397:timestamp)
        n88 = Format Date/Time String(time format string (%c)="%Y", seconds (now)=w397, UTC format=FALSE) -> (date/time string=w389:string)
        n89 = Format Date/Time String(time format string (%c)="%d", seconds (now)=w397, UTC format=FALSE) -> (date/time string=w380:string)
        n90 = call "to_be_2_string.vi"("string 2"=w380) -> ("substring 2"=w379:string)  [unwired: 10 in]
        n91 = Format Date/Time String(time format string (%c)="%m", seconds (now)=w397, UTC format=FALSE) -> (date/time string=w385:string)
        n92 = Concatenate Strings("D" ("磁碟位置"), ":\\LOG運轉紀錄\\", w389, "\\", w385, "\\", w379) -> (w377:string)
        n93 = String To Path(string=w377) -> (path=w393:path)
        n94 = call <vilib>:"Check if File or Folder Exists.vi"("path"=w393) -> ("error out"=w395:errorcluster, "file or folder exists?"=w381:bool, "dup path"=w394:path)  [unwired: 8 in]
        n95 = case shown="False" w381 {
          tunnel: w394 -> [w404 w406]
          tunnel: w395 -> [w403 w405]
          tunnel: [w402 w406] -> _
          tunnel: [w401 w405] -> w378
          frame False {
            n96 = Create Folder(path (use dialog)=w404, error in=w403) -> (created path=w402:path, error out=w401:errorcluster)  [unwired: 1 in, 1 out]
          }
          frame True {
          }
        }
        n97 = Concatenate Strings("explorer ", w377) -> (w399:string)
        n98 = call <vilib>:"System Exec.vi"("wait until completion? (T)"=FALSE, "error in (no error)"=w378, "command line"=w399) -> ()  [unwired: 5 in, 4 out]
      }
      event "Save Button": Value Change {
        n99 = event-data() -> ()  [unwired: 1 in, 6 out]
        n100 = Get Date/Time In Seconds() -> (seconds since 1Jan1904=w436:timestamp)
        n101 = Format Date/Time String(time format string (%c)="%Y", seconds (now)=w436, UTC format=FALSE) -> (date/time string=w417:string)
        n102 = Format Date/Time String(time format string (%c)="%d", seconds (now)=w436, UTC format=FALSE) -> (date/time string=w408:string)
        n103 = call "to_be_2_string.vi"("string 2"=w408) -> ("substring 2"=w407:string)  [unwired: 10 in]
        n104 = Format Date/Time String(time format string (%c)="%m", seconds (now)=w436, UTC format=FALSE) -> (date/time string=w413:string)
        n105 = Format Date/Time String(time format string (%c)="%Y%m%d%H%M%S", seconds (now)=w436) -> (date/time string=w429:string)  [unwired: 1 in]
        n106 = Concatenate Strings("D" ("磁碟位置"), ":\\LOG運轉紀錄\\", w417, "\\", w413, "\\", w407) -> (w424:string)
        n107 = String To Path(string=w424) -> (path=w421:path)
        n108 = call <vilib>:"Check if File or Folder Exists.vi"("path"=w421) -> ("error out"=w423:errorcluster, "file or folder exists?"=w409:bool, "dup path"=w422:path)  [unwired: 8 in]
        n109 = invoke on="Cluster" class="Clust (strict)" method="Get Image"() -> ("image data"=w438:T3)  [unwired: 6 in, 5 out]
        n110 = case shown="False" w409 {
          tunnel: w422 -> [w442 w444]
          tunnel: w423 -> [w441 w443]
          tunnel: [w440 w444] -> w437
          tunnel: [w439 w443] -> _
          frame False {
            n111 = Create Folder(path (use dialog)=w442, error in=w441) -> (created path=w440:path, error out=w439:errorcluster)  [unwired: 1 in, 1 out]
          }
          frame True {
          }
        }
        n112 = Path To String(path=w437) -> (string=w425:string)
        n113 = Concatenate Strings(w425, "\\" ("string"), w429) -> (w435:string)
        n114 = Concatenate Strings(w435, ".jpg" ("file format")) -> (w434:string)
        n115 = String To Path(string=w434) -> (path=w430:path)
        n116 = call <vilib>:"Write JPEG File.vi"("quality (80)"=100, "image data"=w438, "path to JPEG file"=w430) -> ("error out"=→"error out 3":errorcluster)  [unwired: 7 in, 1 out]
      }
    }
    n117 = local read "stop"() -> (w374:bool)
    n118 = Or(x=w373, y=w374) -> (x .or. y?=w369:bool)
    n119 = case shown="True" TRUE {
      tunnel: w369 -> [_ w375]
      frame False {
      }
      frame True {
        n120 = Quit LabVIEW(quit? (T)=w375) -> ()
      }
    }
    "loop2" <- w371
  }
  n121 = local write "stop"(FALSE ("stop")) -> ()
